vi "HighSpeedInit.vi"(6 "timeout":dbl=0.2 format="%#_13g", 8 "error in":errorcluster, 9 "Port":string, 10 "Fast":bool=TRUE, 11 "Python":T1) -> (0 "error out":errorcluster, 3 "Python":T1)   [LabVIEW 2022 SP3]
uses:
  PythonCtrl.ctl
  Processors.ctl
panel:
  out "Console":string
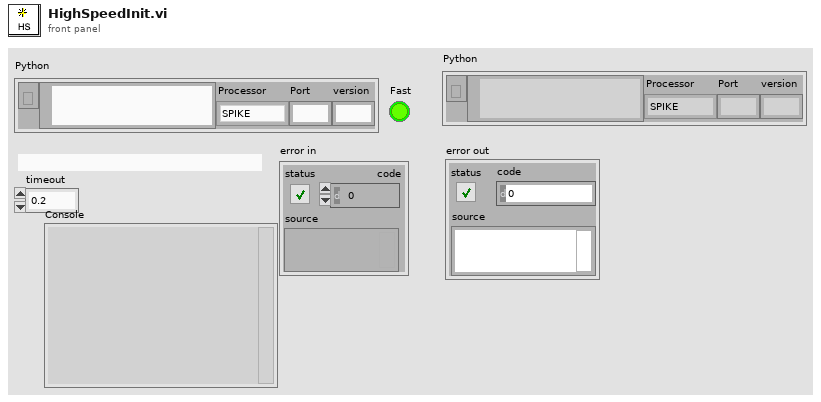
[diagram p1: front panel]
types:
  T1 = typedef "PythonCtrl.ctl" = cluster{"session":refnum<k35>, "PyPath":path, "Processor":T2, "Port":string, "version":string}
  T2 = typedef "Processors.ctl" = enum16{"SPIKE", "Pi", "Pi_ssh", "OpenMV", "Dunio"}
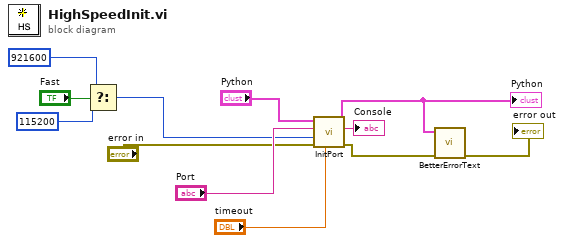
[diagram p0: block diagram]
diagram:
  n1 = Select(t=u32 921600 ("baud rate (115200)"), s="Fast", f=u32 115200 ("baud rate (115200)")) -> (s? t:f=w5:u32)
  n2 = call "InitPort.vi"("timeout"="timeout", "error in (no error)"="error in", "Baud"=w5, "Port"="Port", "Python"="Python") -> ("error out"=w6:errorcluster, "Console"=→"Console":string, "Python out"=w3:T1)  [unwired: 4 in]
  "Python" <- w3
  "error out" <- w6
  n3 = call "BetterErrorText.vi"("error in (no error)"=w6, "Python"=w3) -> ()  [unwired: 8 in, 2 out]
